vi "StandardAttackPlay_Init.vi"(0 "object in":refnum<class "StandardAttackPlay.lvclass">, 5 "error in (no error)":errorcluster) -> (14 "object out":refnum<class "StandardAttackPlay.lvclass">, 19 "error out":errorcluster)   [LabVIEW 2023, in "StandardAttackPlay.lvclass"]
uses:
  StandardAttackPlay.lvclass
  C:/Users/ebert/Documents/codes/SSL/repo/SSL_AI/NewSTP/NewPlays/Play_v2_class/Play_v2.lvclass
  PrimaryAttacker_class/PrimaryAttackerRole.lvclass
  C:/Users/ebert/Documents/codes/SSL/repo/SSL_AI/NewSTP/NewRoles/Role_v2_class/Role_v2.lvclass
  SupportAttackerRole/SupportAttackerRole.lvclass
  Zone_class/zones.ctl
  StandardAttackPlay.lvclass/StandardAttackPlay.ctl
  Zone_class/Zone.lvclass
  Play_v2_class/Play_v2.lvclass
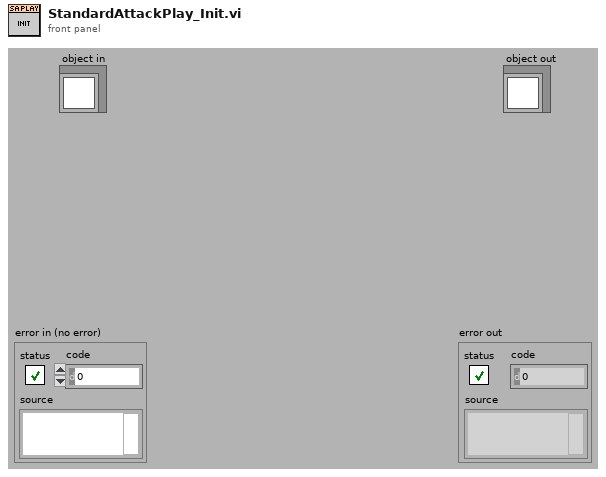
[diagram p1: front panel]
types:
  T1 = typedef "Zone.lvclass/zones.ctl" = enum16{"leftMidField", "rightMidField", "MidField", "leftWing", "rightWing", "LeftSide", "RightSide", "Field", "Size"}
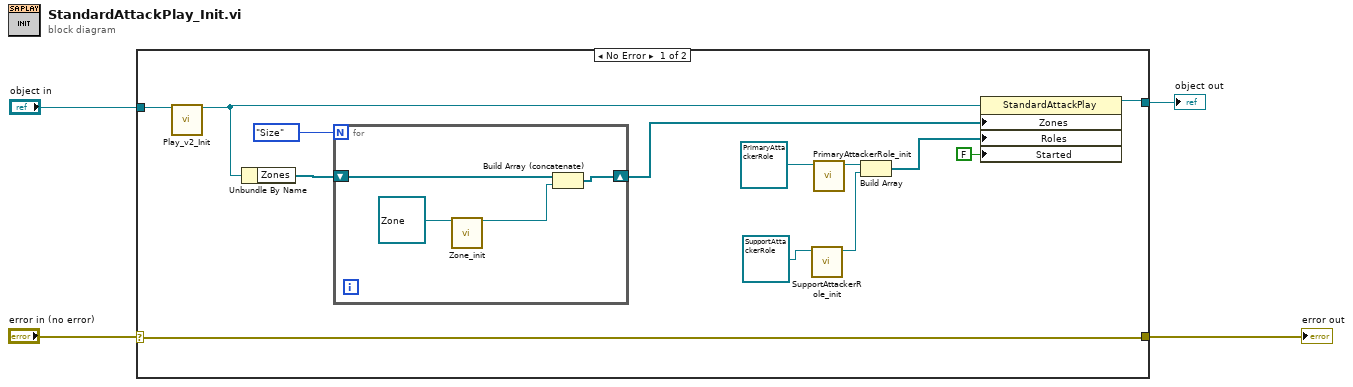
[diagram p0: block diagram]
diagram:
  n1 = case shown="No Error" "error in (no error)" {
    selector: "error in (no error)" -> [w13 w22]
    tunnel: [w16 w23] -> w4
    tunnel: "object in" -> [w17 w23]
    tunnel: [w13 w22] -> w1
    frame No Error {
      n2 = call "Play_v2_Init.vi"("object in"=w17) -> ("object out"=w9:refnum<class "StandardAttackPlay.lvclass">)  [unwired: 17 in, 1 out]
      n3 = Unbundle By Name(w9) -> ("Zones"=w8:refnum<class "Zone.lvclass">[])
      n4 = for {
        N: zones."Size" ("Enum") -> [_]
        shift-right: [w18] -> w6
        shift-left: w8 -> [w21]
        n5 = call "Zone_init.vi"("Zone in"=refnum<class "Zone.lvclass"> refnum ("Zone.lvclass")) -> ("Zone out"=w19:refnum<class "Zone.lvclass">)  [unwired: 17 in, 1 out]
        n6 = Build Array (concatenate)(w21, w19) -> (w18:refnum<class "Zone.lvclass">[])
      }
      n7 = call-dynamic "SupportAttackerRole_init.vi"("SupportAttackerRole in"=refnum<class "SupportAttackerRole.lvclass"> refnum ("SupportAttackerRole.lvclass")) -> ("SupportAttackerRole out"=w10:refnum<class "SupportAttackerRole.lvclass">)  [unwired: 9 in, 1 out]
      n8 = call-dynamic "PrimaryAttackerRole_init.vi"("PrimaryAttackerRole in"=refnum<class "PrimaryAttackerRole.lvclass"> refnum ("PrimaryAttackerRole.lvclass")) -> ("PrimaryAttackerRole out"=w11:refnum<class "PrimaryAttackerRole.lvclass">)  [unwired: 9 in, 1 out]
      n9 = Build Array(w11, w10) -> (w14:refnum<class "Role_v2.lvclass">[])
      n10 = property class="StandardAttackPlay"(reference=w9, "Zones"=w6, "Roles"=w14, "Started"=FALSE) -> (reference out=w16:refnum<class "StandardAttackPlay.lvclass">)  [unwired: 1 in, 1 out]
    }
    frame Error {
    }
  }
  "object out" <- w4
  "error out" <- w1
